vi "PfeifferTC110.vi"(6 "On/off":bool, 7 "Write?":bool, 8 "error in":errorcluster, 9 "Adress":u16=1 max=999 step=1, 10 "VISA session":refnum<visa-resource-name>, 11 "CMD ID":T1) -> (0 "error out":errorcluster, 2 "Response":variant, 3 "VISA session out":refnum<visa-resource-name>)   [LabVIEW 2019]
uses:
  PfeifferTC110Cmds.ctl
  <instrlib>/Pfeiffer Vacuum/Pfeiffer Vacuum.lvlib
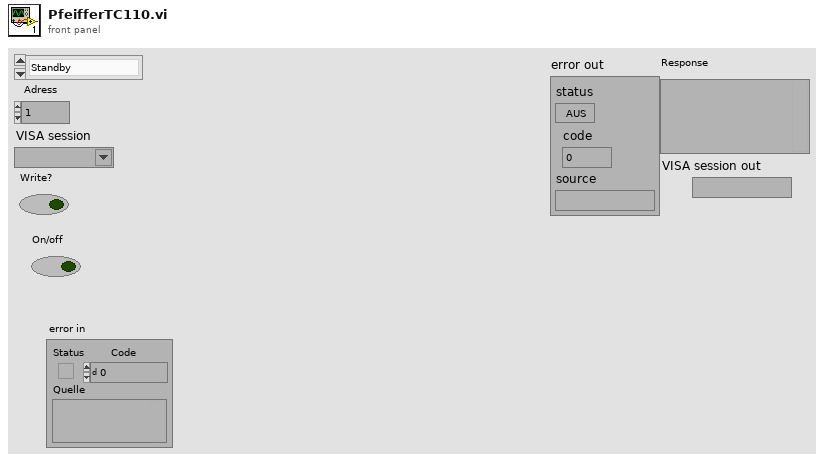
[diagram p1: front panel]
types:
  T1 = typedef "PfeifferTC110Cmds.ctl" = enum16{"Standby", "AckError", "Run", "Motor", "SpdSwPtAtt", "ErrorCode", "OvTempElec", "OvTempPump", "SetSpdAtt", "PumpAccel", "ActualSpdHz", "DrvCurrent", "OpHrsPump", "FwVersion", "DrvVoltage", "OpHrsElec", "NominalSpd", "DrvPower", "PumpCycles", "TempElec", "TempPmpBot", "AccelDecel", "TempBearing", "TempMotor", "ElecName", "HWVersion", "SetRotSpdRPM", "ActualSpdRPM", "NominalSpdRPM"}
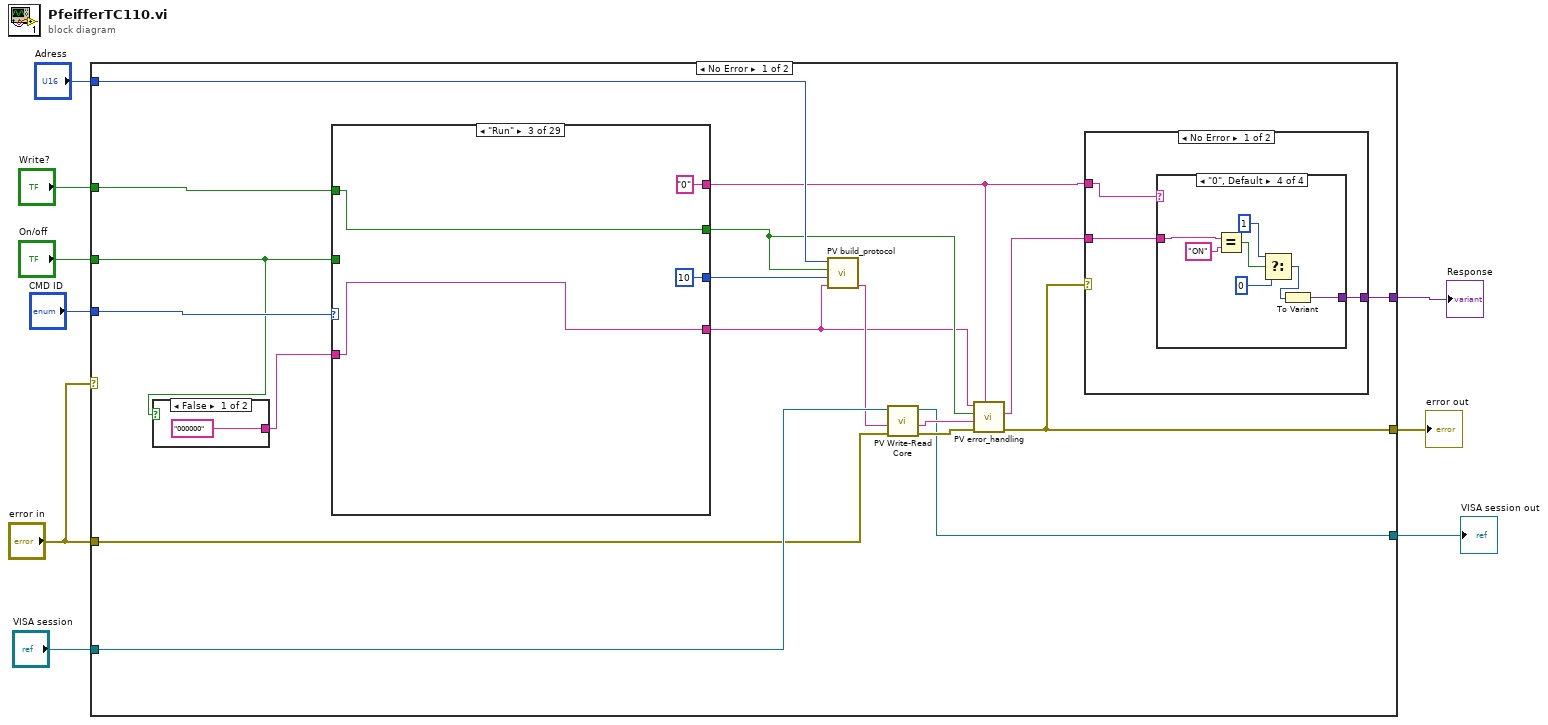
[diagram p0: block diagram]
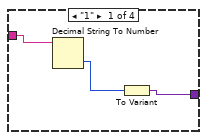
[diagram p2: hidden frame]
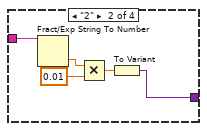
[diagram p3: hidden frame]
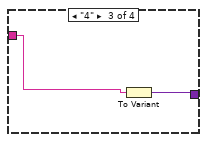
[diagram p4: hidden frame]
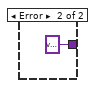
[diagram p5: hidden frame]
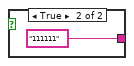
[diagram p6: hidden frame]
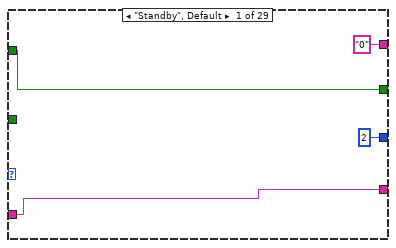
[diagram p7: hidden frame]
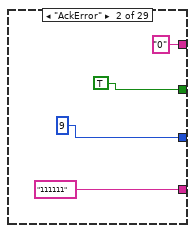
[diagram p8: hidden frame]
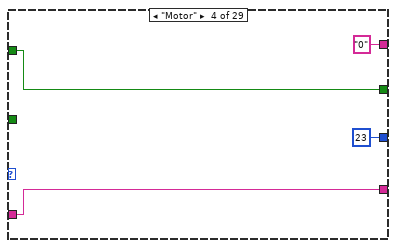
[diagram p9: hidden frame]
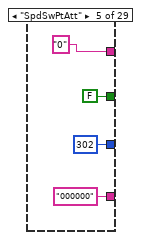
[diagram p10: hidden frame]
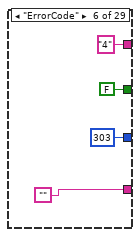
[diagram p11: hidden frame]
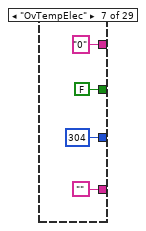
[diagram p12: hidden frame]
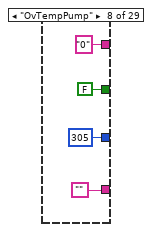
[diagram p13: hidden frame]
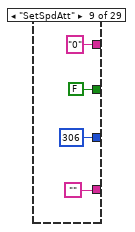
[diagram p14: hidden frame]
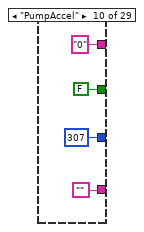
[diagram p15: hidden frame]
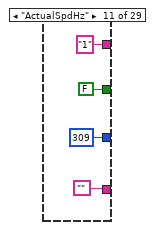
[diagram p16: hidden frame]
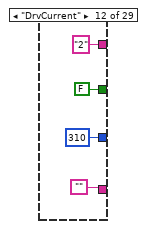
[diagram p17: hidden frame]
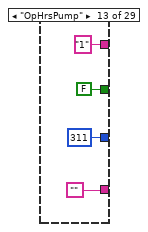
[diagram p18: hidden frame]
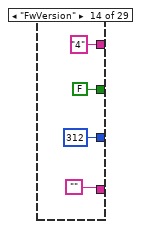
[diagram p19: hidden frame]
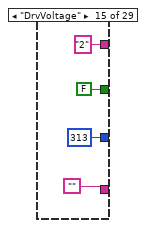
[diagram p20: hidden frame]
diagram:
  n1 = case shown="No Error" "error in" {
    tunnel: "CMD ID" -> [w27 _]
    tunnel: "Adress" -> [w26 _]
    tunnel: "VISA session" -> [w24 w167]
    tunnel: "error in" -> [w22 w169]
    tunnel: "Write?" -> [w21 _]
    tunnel: [w14 w169] -> w5
    tunnel: "On/off" -> [w16 _]
    tunnel: [w11 variant ("Variant")] -> w2
    tunnel: [w10 w167] -> w1
    frame No Error {
      n2 = case shown="False" w16 {
        tunnel: ["000000" ("Data") "111111" ("Data")] -> w15
        frame False {
        }
        frame True {
        }
      }
      n3 = case shown="\"Run\"" w27 {
        tunnel: [u16 2 u16 9 u16 10 u16 23 u16 302 u16 303 u16 304 u16 305 u16 306 u16 307 u16 309 u16 310 u16 311 u16 312 u16 313 u16 314 u16 315 u16 316 u16 319 u16 326 u16 330 u16 336 u16 342 u16 346 u16 349 u16 354 u16 397 u16 398 u16 399] -> w25
        tunnel: [w53 TRUE w62 w65 FALSE ("Write?") FALSE ("Write?") FALSE ("Write?") FALSE ("Write?") FALSE ("Write?") FALSE ("Write?") FALSE ("Write?") FALSE ("Write?") FALSE ("Write?") FALSE ("Write?") FALSE ("Write?") FALSE ("Write?") FALSE ("Write?") FALSE ("Write?") FALSE ("Write?") FALSE ("Write?") FALSE ("Write?") FALSE ("Write?") FALSE ("Write?") FALSE ("Write?") FALSE ("Write?") FALSE ("Write?") FALSE ("Write?") FALSE ("Write?") FALSE ("Write?")] -> w19
        tunnel: [w51 "111111" ("Data") w59 w63 "000000" ("Data") "" "" "" "" "" "" "" "" "" "" "" "" "" "" "" "" "" "" "" "" "" "" "" ""] -> w18
        tunnel: w21 -> [w53 _ w62 w65 _ _ _ _ _ _ _ _ _ _ _ _ _ _ _ _ _ _ _ _ _ _ _ _ _]
        tunnel: w16 -> [_ _ _ _ _ _ _ _ _ _ _ _ _ _ _ _ _ _ _ _ _ _ _ _ _ _ _ _ _]
        tunnel: ["0" "0" "0" "0" "0" "4" "0" "0" "0" "0" "1" "2" "1" "4" "2" "1" "1" "1" "1" "1" "1" "1" "1" "1" "4" "4" "1" "1" "1"] -> w12
        tunnel: w15 -> [w51 _ w59 w63 _ _ _ _ _ _ _ _ _ _ _ _ _ _ _ _ _ _ _ _ _ _ _ _ _]
        frame "Standby", Default {
        }
        frame "AckError" {
        }
        frame "Run" {
        }
        frame "Motor" {
        }
        frame "SpdSwPtAtt" {
        }
        frame "ErrorCode" {
        }
        frame "OvTempElec" {
        }
        frame "OvTempPump" {
        }
        frame "SetSpdAtt" {
        }
        frame "PumpAccel" {
        }
        frame "ActualSpdHz" {
        }
        frame "DrvCurrent" {
        }
        frame "OpHrsPump" {
        }
        frame "FwVersion" {
        }
        frame "DrvVoltage" {
        }
        frame "OpHrsElec" {
        }
        frame "NominalSpd" {
        }
        frame "DrvPower" {
        }
        frame "PumpCycles" {
        }
        frame "TempElec" {
        }
        frame "TempPmpBot" {
        }
        frame "AccelDecel" {
        }
        frame "TempBearing" {
        }
        frame "TempMotor" {
        }
        frame "ElecName" {
        }
        frame "HWVersion" {
        }
        frame "SetRotSpdRPM" {
        }
        frame "ActualSpdRPM" {
        }
        frame "NominalSpdRPM" {
        }
      }
      n4 = call <instrlib>:"PV build_protocol.vi"("Data"=w18, "Parameter-number"=w25, "parameter\nread<->describe"=w19, "Adress"=w26) -> ("output"=w23:string)  [unwired: 3 in]
      n5 = call <instrlib>:"PV Write-Read Core.vi"("error in"=w22, "Write data in"=w23, "VISA session"=w24) -> ("error out"=w17:errorcluster, "response (data) out"=w20:string, "dup VISA session"=w10:refnum<visa-resource-name>)  [unwired: 2 in]
      n6 = call <instrlib>:"PV error_handling.vi"("Data Typ in"=w12, "error in"=w17, "response (data) in"=w20, "Parameter\nread only<->describe"=w19, "data in"=w18) -> ("error out"=w14:errorcluster, "Data out"=w13:string)  [unwired: 4 in, 1 out]
      n7 = case shown="No Error" w14 {
        tunnel: w13 -> [w29 _]
        tunnel: w12 -> [w30 _]
        tunnel: [w28 variant ("Variant")] -> w11
        frame No Error {
          n8 = case shown="\"0\", Default" w30 {
            tunnel: w29 -> [w33 w38 w40 w42]
            tunnel: [w31 w34 w39 w45] -> w28
            frame "1" {
              n9 = Decimal String To Number(string=w33) -> (number=w32:i32)  [unwired: 2 in, 1 out]
              n10 = To Variant(anything=w32) -> (Variant=w31:variant)
            }
            frame "2" {
              n11 = Fract/Exp String To Number(string=w38) -> (number=w37:dbl)  [unwired: 3 in, 1 out]
              n12 = Multiply(x=w37, y=0.01) -> (x*y=w35:dbl)
              n13 = To Variant(anything=w35) -> (Variant=w34:variant)
            }
            frame "4" {
              n14 = To Variant(anything=w40) -> (Variant=w39:variant)
            }
            frame "0", Default {
              n15 = Equal?(x=w42, y="ON") -> (x = y?=w41:bool)
              n16 = Select(t=1, s=w41, f=0) -> (s? t:f=w46:i32)
              n17 = To Variant(anything=w46) -> (Variant=w45:variant)
            }
          }
        }
        frame Error {
        }
      }
    }
    frame Error {
    }
  }
  "error out" <- w5
  "Response" <- w2
  "VISA session out" <- w1
